vi "Conjugate Gradient.vi"(5 "function data":T2, 7 "objective function":T3, 8 "error in (no error)":errorcluster, 9 "stopping criteria":T4={"function tolerance"=1e-06, "parameter tolerance"=1e-06, "max iterations"=100, "max function calls"=1000, "gradient tolerance"=1e-06, "max time (sec)"=-1.0}, 10 "conjugate gradient settings":T1, 11 "start":dbl[](array[numeric])) -> (0 "error out":errorcluster, 1 "number of function evaluations":i32, 2 "f(minimum)":dbl, 3 "minimum":dbl[](array[numeric]))   [LabVIEW 2014, in "NI_Gmath.lvlib"]
doc: "Solves the unconstrained minimization problem for an arbitrary nonlinear function. You must manually select the polymorphic instance to use."
uses:
  NI_Gmath.lvlib
  stopping criteria.ctl
  ucno_user objective function ref.ctl
  objective function data.ctl
  conjugate gradient settings.ctl
  Real Dot Product.vi
  NI_AALBase.lvlib
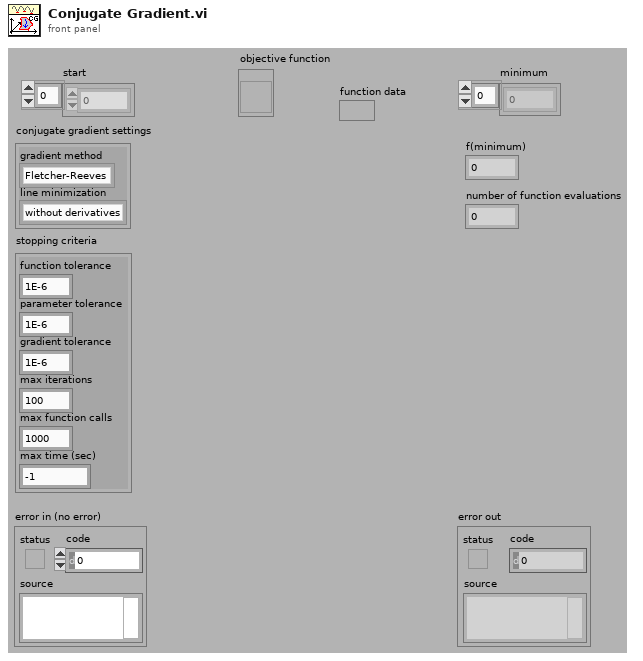
[diagram p1: front panel]
types:
  T1 = typedef "NI_Gmath.lvlib/conjugate gradient settings.ctl" = cluster{"gradient method":enum16{"Fletcher-Reeves", "Polak-Ribiere"}, "line minimization":enum16{"without derivatives", "with derivatives"}}
  T2 = typedef "NI_Gmath.lvlib/objective function data.ctl" = variant
  T3 = typedef "NI_Gmath.lvlib/ucno_user objective function ref.ctl" = refnum<vi>
  T4 = typedef "NI_Gmath.lvlib/stopping criteria.ctl" = cluster{"function tolerance":dbl, "parameter tolerance":dbl, "max iterations":i32, "max function calls":i32, "gradient tolerance":dbl, "max time (sec)":dbl}
  T5 = enum16{"without derivatives", "with derivatives"}
  T6 = cluster{"objective function":T3, "function data":T2}
  T7 = typedef "NI_Gmath.lvlib/stopping criteria with time.ctl" = cluster{"function tolerance":dbl, "parameter tolerance":dbl, "max iterations":i32, "max function calls":i32, "gradient tolerance":dbl, "max time (sec)":dbl, "initial tick count":u32}
  T8 = cluster{"objective function":bool, "gradient":bool}
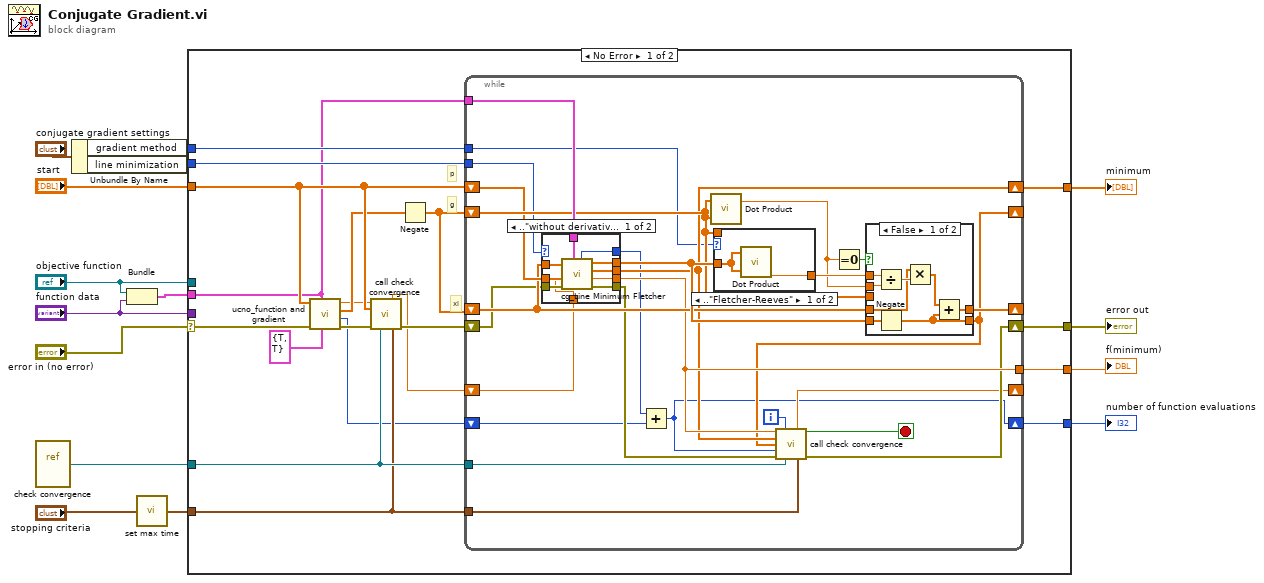
[diagram p0: block diagram]
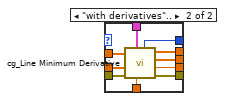
[diagram p2: hidden frame]
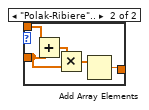
[diagram p3: hidden frame]
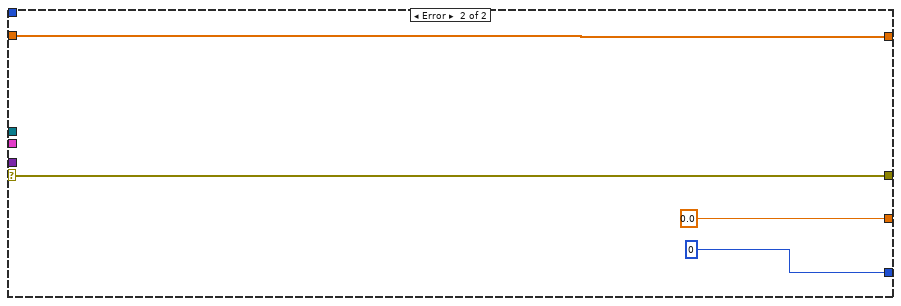
[diagram p5: hidden frame]
diagram:
  n1 = vi-ref "check convergence.vi"() -> ("vi reference"=w9:refnum<vi>)
  n2 = Unbundle By Name("conjugate gradient settings") -> ("gradient method"=w7:enum16{"Fletcher-Reeves", "Polak-Ribiere"}, "line minimization"=w6:T5)
  n3 = Bundle("objective function"="objective function", "function data"="function data") -> (w3:T6)  [unwired: 1 in]
  n4 = call "set max time.vi"("stopping criteria"="stopping criteria") -> ("stopping criteria"=w1:T7)
  n5 = case shown="No Error" "error in (no error)" {
    selector: "error in (no error)" -> [w24 w99]
    tunnel: [w34 w101] -> w15
    tunnel: [w33 0.0 ("f(X)")] -> w14
    tunnel: "start" -> [w23 w101]
    tunnel: "function data" -> [_ _]
    tunnel: "objective function" -> [_ _]
    tunnel: [w26 w99] -> w11
    tunnel: w1 -> [w29 _]
    tunnel: [w16 0 ("number of function evaluations")] -> w10
    tunnel: w9 -> [w30 _]
    tunnel: w7 -> [w28 _]
    tunnel: w6 -> [w27 _]
    tunnel: w3 -> [w18 _]
    frame No Error {
      # "xi"
      # "g"
      # "p"
      n6 = call "ucno_function and gradient.vi"("output control"=T8 {"objective function"=TRUE, "gradient"=TRUE}, "function and data"=w18, "error in (no error)"=w24, "X"=w23) -> ("error out"=w19:errorcluster, "number of function calls"=w17:i32, "gradient"=w21:dbl[], "f(X)"=w20:dbl)  [unwired: 4 in]
      n7 = call "call check convergence.vi"("f"=w20, "X"=w23, "error in"=w19, "vi reference"=w30, "stopping criteria"=w29) -> ("line search tol"=w25:dbl, "error out"=w31:errorcluster)  [unwired: 6 in, 3 out]
      n8 = Negate(x=w21) -> (-x=w32:dbl[])
      n9 = while {
        shift-left: w32 -> [w53]
        shift-right: [w52] -> _
        shift-left: w32 -> [w55]
        shift-right: [w39] -> _
        shift-left: w23 -> [w54]
        shift-right: [w49] -> w34
        shift-right: [w48] -> w26
        shift-left: w31 -> [w51]
        tunnel: w18 -> [w60]
        tunnel: [w50] -> w33
        tunnel: w30 -> [w47]
        tunnel: w29 -> [w46]
        tunnel: w28 -> [w45]
        tunnel: w27 -> [w44]
        shift-right: [w41] -> _
        shift-left: w25 -> [w40]
        shift-right: [w35] -> w16
        shift-left: w17 -> [w36]
        i -> [w43]
        stop <- w42 stop-if-true
        n10 = case shown="..\"without derivatives\"" w44 {
          tunnel: [w70 w80] -> w56
          tunnel: [w66 w76] -> w50
          tunnel: [w67 w79] -> w49
          tunnel: w53 -> [w69 w78]
          tunnel: w54 -> [w68 w77]
          tunnel: [w65 w75] -> w38
          tunnel: w51 -> [w63 w74]
          tunnel: w60 -> [w64 w73]
          tunnel: w40 -> [w62 w72]
          tunnel: [w61 w71] -> w37
          frame .."without derivatives" {
            n11 = call "cg_Line Minimum Fletcher.vi"("function and data"=w64, "error in (no error)"=w63, "tol"=w62, "p"=w68, "xit"=w69) -> ("error out"=w65:errorcluster, "f(p)"=w66:dbl, "pnew"=w67:dbl[], "xitnew"=w70:dbl[], "number of function calls"=w61:i32)  [unwired: 2 in]
          }
          frame "with derivatives".. {
            n12 = call "cg_Line Minimum Derivative.vi"("tol"=w72, "function and data"=w73, "error in (no error)"=w74, "p"=w77, "xit"=w78) -> ("error out"=w75:errorcluster, "f(p)"=w76:dbl, "pnew"=w79:dbl[], "xitnew"=w80:dbl[], "number of function evaluations"=w71:i32)  [unwired: 2 in]
          }
        }
        n13 = Add(x=w37, y=w36) -> (x+y=w35:i32)
        n14 = call-poly "Dot Product.vi"("Y Vector"=w55, "X Vector"=w55) -> ("X * Y"=w57:dbl)  [unwired: 1 out]
        n15 = case shown="..\"Fletcher-Reeves\"" w45 {
          tunnel: w56 -> [w82 w85]
          tunnel: [w81 w83] -> w58
          tunnel: w55 -> [_ w87]
          frame .."Fletcher-Reeves" {
            n16 = call-poly "Dot Product.vi"("Y Vector"=w82, "X Vector"=w82) -> ("X * Y"=w81:dbl)  [unwired: 1 out]
          }
          frame "Polak-Ribiere".. {
            n17 = Add(x=w87, y=w85) -> (x+y=w86:dbl[])
            n18 = Multiply(x=w86, y=w85) -> (x*y=w84:dbl[])
            n19 = Add Array Elements(numeric array=w84) -> (sum=w83:dbl)
          }
        }
        n20 = Equal To 0?(x=w57) -> (x = 0?=w59:bool)
        n21 = case shown="False" w59 {
          tunnel: w57 -> [w95 _]
          tunnel: w58 -> [w94 _]
          tunnel: w53 -> [w92 w97]
          tunnel: w56 -> [w91 _]
          tunnel: [w90 w96] -> w39
          tunnel: [w88 w97] -> w52
          tunnel: w55 -> [_ w96]
          frame False {
            n22 = Divide(x=w94, y=w95) -> (x/y=w93:dbl)
            n23 = Negate(x=w91) -> (-x=w90:dbl[])
            n24 = Multiply(x=w92, y=w93) -> (x*y=w89:dbl[])
            n25 = Add(x=w89, y=w90) -> (x+y=w88:dbl[])
          }
          frame True {
          }
        }
        n26 = call "call check convergence.vi"("f"=w50, "current iteration"=w43, "X"=w49, "gradient"=w39, "number of function evaluations"=w35, "error in"=w38, "vi reference"=w47, "stopping criteria"=w46) -> ("line search tol"=w41:dbl, "stop?"=w42:bool, "error out"=w48:errorcluster)  [unwired: 3 in, 2 out]
      }
    }
    frame Error {
    }
  }
  "f(minimum)" <- w14
  "minimum" <- w15
  "error out" <- w11
  "number of function evaluations" <- w10
